vi "FOCUS_V42_H37.vi"(9 "X-pixels":sgl=256.0, 11 "Run":bool) -> (0 "Retrace pixels":sgl, 10 "Pixel Clock (Hz)":sgl)   [LabVIEW 2010] (continued)
                      tunnel: w5384 -> [w5402 w5420]
                      tunnel: w5353 -> [w5401 w5419]
                      tunnel: [w5400 w5418] -> w5383
                      tunnel: [w5399 w5417] -> w5382
                      tunnel: [w5399 w5417] -> w5369
                      tunnel: w5368 -> [_ _]
                      tunnel: w5361 -> [w5398 _]
                      tunnel: w5360 -> [w5394 w5415]
                      tunnel: [w5396 w5413] -> w5342
                      tunnel: w5341 -> [w5395 _]
                      frame False {
                        n2973 = case shown="True" w5395 {
                          tunnel: [w5403 w5404] -> w5396
                          tunnel: w5394 -> [w5403 _]
                          frame False {
                          }
                          frame True {
                            n2974 = local read "scattering length [µm]"() -> (w5412:sgl)
                            n2975 = local read "z-step (um)"() -> (w5408:sgl)
                            n2976 = Divide(x=w5408, y=w5412) -> (x/y=w5409:sgl)
                            n2977 = Exponential(1:w5409) -> (0:w5410:sgl)
                            n2978 = local read "Intensity"() -> (w5411:sgl)
                            n2979 = local read "IntensityScaleMax"() -> (w5405:sgl)
                            n2980 = Multiply(x=w5411, y=w5410) -> (x*y=w5406:sgl)
                            n2981 = In Range and Coerce(upper limit=sgl 0.0, x=w5406, lower limit=w5405) -> (coerced(x)=w5404:sgl)  [unwired: 1 out]
                            n2982 = local write "Intensity"(w5404) -> ()
                          }
                        }
                        n2983 = Build Array(w5398, w5396) -> (w5397:dbl[])
                        n2984 = call-poly <vilib>:"DAQmx Write (Analog 1D DBL NChan 1Samp).vi"("task/channels in"=w5402, "data"=w5397, "error in"=w5401) -> ("task out"=w5399:refnum<k21>, "error out"=w5400:errorcluster)  [unwired: 10 in, 1 out]
                      }
                      frame True {
                        n2985 = local read "IntensityScaleMax"() -> (w5414:sgl)
                        n2986 = In Range and Coerce(upper limit=sgl 0.0, x=w5415, lower limit=w5414) -> (coerced(x)=w5413:sgl)  [unwired: 1 out]
                        n2987 = local write "Intensity"(w5413) -> ()
                        n2988 = Build Array(0.0 ("data"), w5413) -> (w5422:dbl[])
                        n2989 = call-poly <vilib>:"DAQmx Write (Analog 1D DBL NChan 1Samp).vi"("task/channels in"=w5420, "data"=w5422, "error in"=w5419) -> ("task out"=w5417:refnum<k21>, "error out"=w5418:errorcluster)  [unwired: 10 in, 1 out]
                      }
                    }
                    n2990 = case shown="False" w5327 {
                      tunnel: [w5432 w5458] -> w5372
                      tunnel: [w5431 w5457] -> w5371
                      tunnel: [w5429 w5455] -> w5357
                      tunnel: w5370 -> [w5428 w5458]
                      tunnel: w5369 -> [w5427 _]
                      tunnel: w5368 -> [w5426 w5457]
                      tunnel: w5359 -> [w5425 w5456]
                      tunnel: [w5424 w5456] -> w5358
                      tunnel: w5363 -> [w5423 w5455]
                      frame False {
                        n2991 = flat-sequence {
                          tunnel: sgl 100.0 ("Time interval [s]") -> [w5444]
                          tunnel: [w5444] -> w5438
                          tunnel: [w5440] -> w5437
                          tunnel: [w5439] -> w5436
                          tunnel: w5428 -> [w5442]
                          tunnel: w5426 -> [w5441]
                          tunnel: [w5451] -> w5435
                          tunnel: [w5450] -> w5434
                          tunnel: [w5449] -> w5433
                          tunnel: w5438 -> [w5451]
                          tunnel: w5437 -> [w5450]
                          tunnel: w5436 -> [w5449]
                          tunnel: w5425 -> [w5448]
                          tunnel: w5423 -> [w5447]
                          tunnel: [w5446] -> w5429
                          tunnel: [w5445] -> w5424
                          tunnel: [w5454] -> w5432
                          tunnel: w5435 -> [w5453]
                          tunnel: w5434 -> [w5454]
                          tunnel: w5433 -> [w5452]
                          tunnel: [w5452] -> w5431
                          tunnel: w5427 -> [_]
                          frame #0 {
                            w5443 = FALSE ("data")
                            n2992 = local write "Shutter open"(w5443) -> ()
                            n2993 = call-poly <vilib>:"DAQmx Write (Digital Bool 1Line 1Point).vi"("task/channels in"=w5442, "data"=w5443, "error in"=w5441) -> ("task out"=w5440:refnum<k21>, "error out"=w5439:errorcluster)  [unwired: 10 in, 1 out]
                          }
                          frame #1 {
                            n2994 = call <vilib>:"DAQmx Stop Task.vi"("task/channels in"=w5448, "error in"=w5447) -> ("task out"=w5445:refnum<k21>, "error out"=w5446:errorcluster)  [unwired: 12 in]
                          }
                          frame #2 {
                            n2995 = Wait (ms)(milliseconds to wait=w5453) -> ()  [unwired: 1 out]
                          }
                        }
                      }
                      frame True {
                      }
                    }
                    n2996 = call "ConvertImagesDataFOCUS.vi"("Save mode"=w5321, "Image3"=w5325, "Image2"=w5334, "Image1"=w5335) -> ("Data"=w5333:u8[])
                    n2997 = Set File Position(refnum=w5339, from (0:start)=enum16{"start", "end", "current"}."current" ("pos mode (0:2)"), error in=w5338) -> (refnum out=w5320:refnum<file>, error out=w5319:errorcluster)  [unwired: 1 in]
                    n2998 = Write to Binary File(file (use dialog)=w5320, data=w5333, error in=w5319, 5:FALSE ("prepend array or string size? (T)")) -> (refnum out=w5337:refnum<file>, error out=w5336:errorcluster)  [unwired: 2 in, 1 out]
                    n2999 = local read "Y-lines"() -> (w5381:sgl)
                    n3000 = Multiply(x=w5354, y=w5381) -> (x*y=w5379:sgl)
                    n3001 = Replace Array Subset(array=w5386, new element=w5335, index (row)=0 ("disabled index (row)"), index (col)=w5379) -> (w5385:u8[][])
                    n3002 = Replace Array Subset(array=w5388, new element=w5334, index (row)=0 ("disabled index (row)"), index (col)=w5379) -> (w5387:u8[][])
                  }
                  n3003 = Not Equal?(x=w5254, y=w5255) -> (x != y?=w5256:bool)
                  n3004 = local write "IntDevUsed"(w5256) -> ()
                  n3005 = Close File(refnum=w5241, error in=w5240) -> ()  [unwired: 2 out]
                  n3006 = flat-sequence {
                    tunnel: [w5303] -> w5265
                    tunnel: w5267 -> [w5303]
                    tunnel: w5266 -> [w5302]
                    tunnel: [w5302] -> w5264
                    frame #0 {
                      n3007 = Tick Count (ms)() -> (millisecond timer value=w5304:u32)
                      n3008 = local write "stop"(w5304) -> ()
                    }
                  }
                }
                frame 5 {
                  w5745 = sgl 1000000.0 ("y")
                  w5777 = 0.0 ("X Scale.Range:Minimum")
                  w5784 = TRUE ("Visible")
                  # "User-defined line 3D"
                  n3009 = Greater Or Equal?(x=w5711, y=u16 3) -> (x >= y?=w5709:bool)
                  n3010 = property on="Property Node" class="VI"() -> ("VI Path"=w5739:path)  [unwired: 2 in, 2 out]
                  n3011 = property on="Property Node" class="VI"() -> ("VI Path"=w5720:path)  [unwired: 2 in, 2 out]
                  n3012 = flat-sequence {
                    tunnel: w5786 -> [w5801]
                    tunnel: [w5801] -> w5785
                    frame #0 {
                      n3013 = Tick Count (ms)() -> (millisecond timer value=w5802:u32)
                      n3014 = local write "start"(w5802) -> ()
                    }
                  }
                  n3015 = Unbundle By Name(w5724) -> ("status"=w5758:bool)
                  n3016 = Increment(x=w5735) -> (x+1=w5734:sgl)
                  n3017 = Tick Count (ms)() -> (millisecond timer value=w5790:u32)
                  n3018 = Strip Path(path=w5739) -> (stripped path=w5738:path)  [unwired: 1 out]
                  n3019 = Strip Path(path=w5720) -> (stripped path=w5719:path)  [unwired: 1 out]
                  n3020 = local read "X-pixels FreeLine"() -> (w5744:sgl)
                  n3021 = local read "Y-lines FreeLine"() -> (w5746:sgl)
                  n3022 = Build Path(base path=w5738, name or relative path="FreeLine.tmp") -> (appended path=w5737:path)
                  n3023 = Build Path(base path=w5719, name or relative path="EEG.tmp") -> (appended path=w5718:path)
                  n3024 = call <vilib>:"Open_Create_Replace File.vi"("advisory dialog? (display:T)"=FALSE, "function (open:0)"=T8."create or replace", "file path"=w5737) -> ("error out"=w5728:errorcluster, "refnum"=w5730:refnum<file>)  [unwired: 5 in, 2 out]
                  n3025 = Unbundle By Name(w5760) -> ("status"=w5759:bool)
                  n3026 = call <vilib>:"Open_Create_Replace File.vi"("advisory dialog? (display:T)"=FALSE, "function (open:0)"=T8."create or replace", "file path"=w5718) -> ("error out"=w5716:errorcluster, "refnum"=w5715:refnum<file>)  [unwired: 5 in, 2 out]
                  n3027 = Divide(x=w5745, y=w5744) -> (x/y=w5743:sgl)
                  n3028 = Multiply(x=w5746, y=w5744) -> (x*y=w5747:sgl)
                  n3029 = local read "XScale"() -> (w5778:bool)
                  n3030 = Greater?(x=w5747, y=w5745) -> (0:w5748:bool)
                  n3031 = Select(t=w5743, s=w5748, f=w5746) -> (s? t:f=w5742:sgl)
                  n3032 = case shown="True" w5778 {
                    tunnel: [w5797 w5798] -> w5776
                    tunnel: w5742 -> [w5797 _]
                    tunnel: w5744 -> [_ w5798]
                    frame False {
                    }
                    frame True {
                    }
                  }
                  n3033 = Set File Position(refnum=w5730, from (0:start)=enum16{"start", "end", "current"}."start" ("pos mode (rel. to end:1)"), error in=w5728) -> (refnum out=w5708:refnum<file>, error out=w5707:errorcluster)  [unwired: 1 in]
                  n3034 = Write to Binary File(file (use dialog)=w5708, data=w5731, error in=w5707, 5:FALSE ("prepend array or string size? (T)")) -> (refnum out=w5729:refnum<file>, error out=w5727:errorcluster)  [unwired: 2 in, 1 out]
                  n3035 = while {
                    tunnel: [w5842] -> w5791
                    tunnel: [w5840] -> w5788
                    tunnel: w5792 -> [w5871]
                    tunnel: w5785 -> [w5864]
                    shift-right: [w5847] -> w5752
                    shift-left: w5793 -> [w5903]
                    tunnel: w5749 -> [w5818]
                    shift-right: [w5849] -> w5753
                    shift-left: w5793 -> [w5902]
                    shift-right: [w5897] -> _
                    shift-left: w5790 -> [w5898]
                    tunnel: w5782 -> [w5874]
                    tunnel: w5781 -> [w5865]
                    tunnel: [w5873] -> w5779
                    tunnel: [w5872] -> w5780
                    shift-right: [w5877] -> w5733
                    shift-left: w5775 -> [w5879]
                    tunnel: w5765 -> [w5875]
                    tunnel: w5764 -> [w5863]
                    tunnel: [w5875] -> w5762
                    tunnel: [w5863] -> w5763
                    tunnel: [w5867] -> w5761
                    tunnel: w5759 -> [w5862]
                    tunnel: w5758 -> [w5858]
                    shift-right: [w5851] -> w5750
                    shift-left: w5729 -> [w5853]
                    shift-right: [w5850] -> w5751
                    shift-left: w5727 -> [w5852]
                    tunnel: w5734 -> [w5844]
                    tunnel: w5726 -> [w5838]
                    tunnel: w5724 -> [w5837]
                    tunnel: [w5836] -> w5725
                    tunnel: [w5835] -> w5723
                    shift-right: [w5827] -> w5714
                    shift-left: w5715 -> [w5829]
                    shift-right: [w5826] -> w5713
                    shift-left: w5716 -> [w5828]
                    tunnel: w5712 -> [w5824]
                    tunnel: w5711 -> [w5814]
                    tunnel: w5709 -> [w5809]
                    i -> [w5845]
                    stop <- w5854 stop-if-true
                    # "DIO Read reads one\nline of data at a time"
                    n3036 = Unbundle By Name(w5863) -> ("status"=w5861:bool)
                    n3037 = Unbundle By Name(w5865) -> ("status"=w5860:bool)
                    n3038 = Equal To 0?(x=w5845) -> (x = 0?=w5884:bool)
                    n3039 = Unbundle By Name(w5864) -> ("status"=w5859:bool)
                    n3040 = local read "End experiment"() -> (w5856:bool)
                    n3041 = local read "Y-lines FreeLine"() -> (w5866:sgl)
                    n3042 = case shown="False" w5884 {
                      tunnel: w5818 -> [w5963 w5966]
                      tunnel: [w5963 w5965] -> w5817
                      tunnel: w5824 -> [_ w5964]
                      tunnel: [sgl 0.0 w5964] -> w5819
                      frame False {
                      }
                      frame True {
                        n3043 = Add(x=w5966, y=w5964) -> (x+y=w5965:sgl)
                      }
                    }
                    n3044 = call-poly <vilib>:"DAQmx Read (Analog 2D DBL NChan NSamp).vi"("task/channels in"=w5874, "number of samples per channel"=w5817, "error in"=w5865) -> ("task out"=w5873:refnum<k21>, "data"=w5821:dbl[][], "error out"=w5872:errorcluster)  [unwired: 10 in]
                    n3045 = Array Subset(array=w5821, index (col)=w5819) -> (w5820:dbl[][])  [unwired: 3 in]
                    n3046 = local read "stop 2"() -> (w5857:bool)
                    n3047 = Transpose 2D Array(2D array=w5820) -> (transposed array=w5831:dbl[][])
                    n3048 = Increment(x=w5845) -> (x+1=w5876:i32)
                    n3049 = call-poly <vilib>:"DAQmx Read (Digital 1D U32 1Chan NSamp).vi"("task/channels in"=w5871, "number of samples per channel"=w5817, "error in"=w5864) -> ("task out"=w5843:refnum<k21>, "data"=w5823:u32[], "error out"=w5841:errorcluster)  [unwired: 10 in]
                    n3050 = Build Array (concatenate)(w5879, w5831) -> (w5878:dbl[][])
                    n3051 = Multiply(x="z frequency", y=w5818) -> (x*y=w5834:dbl)
                    n3052 = Index Array(array=w5831, index (col)=0 ("disabled index (col)")) -> (element=w5881:dbl[])  [unwired: 1 in]
                    n3053 = Equal?(x=w5876, y=w5866) -> (x = y?=w5855:bool)
                    n3054 = local write "#"(w5876) -> ()
                    n3055 = Index Array(array=w5831, index (col)=1 ("disabled index (col)")) -> (element=w5880:dbl[])  [unwired: 1 in]
                    n3056 = Array Subset "Extract DI0"(array=w5823, index=w5819) -> (w5822:u32[])  [unwired: 1 in]
                    n3057 = Index Array(array=w5831, index (col)=3 ("disabled index (col)")) -> (element=w5825:dbl[])  [unwired: 1 in]
                    n3058 = local read "Overlay Images"() -> (w5885:bool)
                    n3059 = property class="DAQmx Timing"(reference=w5838, error in=w5837, "Sample Clock:Rate"=w5834) -> (reference out=w5836:refnum<k21>, error out=w5835:errorcluster)
                    n3060 = Compound Arithmetic op=OR(w5855, w5856, w5857, w5858, w5859, w5860, w5861, w5862) -> (w5854:bool)
                    n3061 = Array Subset(array=w5878, index (row)=w5818) -> (w5877:dbl[][])  [unwired: 3 in]
                    n3062 = local read "x scale"() -> (w5891:dbl)
                    n3063 = local read "y scale"() -> (w5889:dbl)
                    n3064 = Split Number(x=w5822) -> (hi(x)=w5816:u16[], lo(x)=w5815:u16[])
                    n3065 = property class="DAQmx Read"(reference=w5843, error in=w5841) -> (reference out=w5842:refnum<k21>, error out=w5840:errorcluster, "Status:Available Samples Per Channel"=→"Scan Backlock":u32)
                    n3066 = case shown="0, Default" w5814 {
                      tunnel: w5816 -> [w5915 w5920 w5925 w5930 w5935 w5940]
                      tunnel: [w5914 w5919 w5922 w5929 w5934 w5937] -> w5813
                      tunnel: [w5912 w5917 w5924 w5927 w5932 w5939] -> w5812
                      tunnel: w5815 -> [w5913 w5918 w5923 w5928 w5933 w5938]
                      tunnel: [w5911 w5916 w5921 w5926 w5931 w5936] -> w5811
                      frame 0, Default {
                        n3067 = Split Number(x=w5915) -> (hi(x)=w5914:u8[], lo(x)=w5912:u8[])
                        n3068 = Split Number(x=w5913) -> (lo(x)=w5911:u8[])  [unwired: 1 out]
                      }
                      frame 1 {
                        n3069 = Split Number(x=w5920) -> (hi(x)=w5919:u8[], lo(x)=w5916:u8[])
                        n3070 = Split Number(x=w5918) -> (lo(x)=w5917:u8[])  [unwired: 1 out]
                      }
                      frame 2 {
                        n3071 = Split Number(x=w5925) -> (hi(x)=w5921:u8[], lo(x)=w5924:u8[])
                        n3072 = Split Number(x=w5923) -> (lo(x)=w5922:u8[])  [unwired: 1 out]
                      }
                      frame 3 {
                        n3073 = Split Number(x=w5930) -> (hi(x)=w5929:u8[], lo(x)=w5927:u8[])
                        n3074 = Split Number(x=w5928) -> (lo(x)=w5926:u8[])  [unwired: 1 out]
                      }
                      frame 4 {
                        n3075 = Split Number(x=w5935) -> (hi(x)=w5934:u8[], lo(x)=w5931:u8[])
                        n3076 = Split Number(x=w5933) -> (lo(x)=w5932:u8[])  [unwired: 1 out]
                      }
                      frame 5 {
                        n3077 = Split Number(x=w5940) -> (hi(x)=w5936:u8[], lo(x)=w5939:u8[])
                        n3078 = Split Number(x=w5938) -> (lo(x)=w5937:u8[])  [unwired: 1 out]
                      }
                    }
                    n3079 = Tick Count (ms)() -> (millisecond timer value=w5899:u32)
                    n3080 = Multiply(x=w5880, y=w5889) -> (x*y=w5893:dbl[])
                    n3081 = Multiply(x=w5891, y=w5881) -> (x*y=w5895:dbl[])
                    n3082 = local read "x offset"() -> (w5890:dbl)
                    n3083 = case shown="True" w5885 {
                      tunnel: w5813 -> [w5968 w5971]
                      tunnel: [w5968 w5969] -> w5887
                      tunnel: w5812 -> [w5967 w5970]
                      tunnel: [w5967 _] -> w5886
                      frame False {
                      }
                      frame True {
                        n3084 = To Word Integer(number=w5971) -> (16bit integer=w5976:i16[])
                        n3085 = Subtract(x=w5976, y=w5970) -> (x-y=w5977:i16[])
                        n3086 = Add(x=w5976, y=w5970) -> (x+y=w5981:i16[])
                        n3087 = Increment(x=w5981) -> (x+1=w5972:i16[])
                        n3088 = Divide(x=w5977, y=w5972) -> (x/y=w5973:dbl[])
                        n3089 = Absolute Value(x=w5977) -> (abs(x)=w5979:i16[])
                        n3090 = Multiply(x=w5973, y=u8 2) -> (x*y=w5975:dbl[])
                        n3091 = Round To Nearest(number=w5975) -> (nearest integer value=w5988:dbl[])
                        n3092 = Divide(x=w5979, y=2.0) -> (x/y=w5982:dbl[])
                        n3093 = Divide(x=w5981, y=2.0) -> (x/y=w5983:dbl[])
                        n3094 = Add(x=w5982, y=w5983) -> (x+y=w5985:dbl[])
                        n3095 = Divide(x=w5985, y=5.0) -> (x/y=w5986:dbl[])
                        n3096 = Round To Nearest(number=w5986) -> (nearest integer value=w5987:dbl[])
                        n3097 = Multiply(x=5.0 ("y"), y=w5987) -> (x*y=w5989:dbl[])
                        n3098 = Add(x=w5988, y=w5989) -> (x+y=w5990:dbl[])
                        n3099 = Subtract(x=w5990, y=2.0) -> (x-y=w5993:dbl[])
                        n3100 = To Unsigned Byte Integer(number=w5993) -> (unsigned 8bit integer=w5969:u8[])
                      }
                    }
                    n3101 = Subtract(x=w5899, y=w5898) -> (x-y=w5900:u32)
                    n3102 = local read "y offset"() -> (w5888:dbl)
                    n3103 = local read "Image Update [ms]"() -> (w5870:u32)
                    n3104 = Add(x=w5893, y=w5888) -> (x+y=w5892:dbl[])
                    n3105 = Add(x=w5890, y=w5895) -> (x+y=w5894:dbl[])
                    n3106 = Subtract(x=w5845, y=w5818) -> (x-y=w5867:sgl)
                    n3107 = case shown="True" w5809 {
                      tunnel: w5813 -> [w5907 w5910]
                      tunnel: w5812 -> [w5904 w5909]
                      tunnel: w5811 -> [w5906 _]
                      tunnel: [w5905 w5908] -> w5810
                      frame True {
                        n3108 = Interleave 1D Arrays(w5904, w5907, w5906) -> (w5905:u8[])
                      }
                      frame False {
                        n3109 = Interleave 1D Arrays(w5910, w5909) -> (w5908:u8[])
                      }
                    }
                    n3110 = Multiply(x=w5870, y=u32 20) -> (x*y=w5868:u32)
                    n3111 = Greater Or Equal?(x=w5900, y=w5868) -> (x >= y?=w5901:bool)
                    n3112 = Greater Or Equal?(x=w5845, y=w5844) -> (x >= y?=w5846:bool)
                    n3113 = case shown="True" w5846 {
                      tunnel: w5903 -> [w5947 w5960]
                      tunnel: w5902 -> [w5946 w5954]
                      tunnel: w5887 -> [w5945 w5958]
                      tunnel: w5886 -> [w5944 w5951]
                      tunnel: [w5943 w5948] -> w5849
                      tunnel: [w5942 w5961] -> w5847
                      tunnel: w5845 -> [w5941 _]
                      frame False {
                        n3114 = Replace Array Subset(array=w5947, new element=w5945, index (col)=w5941) -> (w5942:u8[][])  [unwired: 1 in]
                        n3115 = Replace Array Subset(array=w5946, new element=w5944, index (col)=w5941) -> (w5943:u8[][])  [unwired: 1 in]
                      }
                      frame True {
                        n3116 = Transpose 2D Array(2D array=w5954) -> (transposed array=w5952:u8[][])
                        n3117 = Transpose 2D Array(2D array=w5960) -> (transposed array=w5959:u8[][])
                        n3118 = Build Array (concatenate)(w5952, w5951) -> (w5953:u8[][])
                        n3119 = Build Array (concatenate)(w5959, w5958) -> (w5957:u8[][])
                        n3120 = Transpose 2D Array(2D array=w5953) -> (transposed array=w5949:u8[][])
                        n3121 = Transpose 2D Array(2D array=w5957) -> (transposed array=w5956:u8[][])
                        n3122 = Array Subset(array=w5956, index (col)=1 ("index")) -> (w5961:u8[][])  [unwired: 3 in]
                        n3123 = Array Subset(array=w5949, index (col)=1 ("index")) -> (w5948:u8[][])  [unwired: 3 in]
                      }
                    }
                    n3124 = Set File Position(refnum=w5829, from (0:start)=enum16{"start", "end", "current"}."current" ("pos mode (0:2)"), error in=w5828) -> (refnum out=w5808:refnum<file>, error out=w5807:errorcluster)  [unwired: 1 in]
                    n3125 = Write to Binary File(file (use dialog)=w5808, data=w5825, error in=w5807, 5:FALSE ("prepend array or string size? (T)")) -> (refnum out=w5827:refnum<file>, error out=w5826:errorcluster)  [unwired: 2 in, 1 out]
                    n3126 = Set File Position(refnum=w5853, from (0:start)=enum16{"start", "end", "current"}."current" ("pos mode (0:2)"), error in=w5852) -> (refnum out=w5805:refnum<file>, error out=w5804:errorcluster)  [unwired: 1 in]
                    n3127 = Write to Binary File(file (use dialog)=w5805, data=w5810, error in=w5804, 5:FALSE ("prepend array or string size? (T)")) -> (refnum out=w5851:refnum<file>, error out=w5850:errorcluster)  [unwired: 2 in, 1 out]
                    n3128 = Bundle(w5894, w5892) -> (w5896:cluster{dbl[], dbl[]})  [unwired: 1 in]
                    n3129 = case shown="True" w5901 {
                      tunnel: [w5994 w5998] -> w5897
                      tunnel: w5898 -> [w5994 _]
                      tunnel: w5896 -> [_ w5997]
                      tunnel: w5847 -> [_ w5996]
                      tunnel: w5849 -> [_ w5995]
                      frame False {
                      }
                      frame True {
                        n3130 = local write "XY Graph 3"(w5997) -> ()
                        n3131 = local write "XY Graph 4"(w5997) -> ()
                        n3132 = local write "Image 4"(w5995) -> ()
                        n3133 = local write "Image 3"(w5996) -> ()
                        n3134 = Tick Count (ms)() -> (millisecond timer value=w5998:u32)
                      }
                    }
                  }
                  n3135 = property on="Image 2" class="IntGraph (strict)"() -> ("Color Table"=w5783:u32[])  [unwired: 2 in, 2 out]
                  n3136 = property on="Image 3" class="IntGraph (strict)"("X Scale.Range:Minimum"=w5777, "X Scale.Range:Maximum"=w5776, "Y Scale.Range:Minimum"=w5777, "Y Scale.Range:Maximum"=w5742, "Visible"=w5784, "Color Table"=w5783) -> ()  [unwired: 2 in, 2 out]
                  n3137 = property on="Image 4" class="IntGraph (strict)"("X Scale.Range:Minimum"=w5777, "X Scale.Range:Maximum"=w5776, "Y Scale.Range:Minimum"=w5777, "Y Scale.Range:Maximum"=w5742, "Visible"=w5784, "Color Table"=w5783) -> ()  [unwired: 2 in, 2 out]
                  n3138 = property on="Histogram1" class="XYGraph (strict)"("X Scale.Range:Minimum"=w5777, "X Scale.Range:Maximum"=w5776) -> ()  [unwired: 2 in, 2 out]
                  n3139 = property on="Histogram2" class="XYGraph (strict)"("X Scale.Range:Minimum"=w5777, "X Scale.Range:Maximum"=w5776) -> ()  [unwired: 2 in, 2 out]
                  n3140 = Close File(refnum=w5750, error in=w5751) -> ()  [unwired: 2 out]
                  n3141 = Close File(refnum=w5714, error in=w5713) -> ()  [unwired: 2 out]
                  n3142 = Array Subset(array=w5733, index (col)=0 ("index"), length (col)=3 ("length")) -> (w5766:dbl[][])  [unwired: 2 in]
                  n3143 = Index Array(array=w5766, index (col)=0 ("disabled index (col)")) -> (element=w5773:dbl[])  [unwired: 1 in]
                  n3144 = flat-sequence {
                    tunnel: w5788 -> [w5799]
                    tunnel: [w5799] -> w5787
                    frame #0 {
                      n3145 = Tick Count (ms)() -> (millisecond timer value=w5800:u32)
                      n3146 = local write "stop"(w5800) -> ()
                    }
                  }
                  n3147 = Array Size(array=w5773) -> (size(s)=w5772:i32)
                  n3148 = Multiply(x=w5772, y=3) -> (x*y=w5770:i32)
                  n3149 = Reshape Array(w5766, w5770) -> (w5769:dbl[])
                  n3150 = local write "Positions"(w5769) -> ()
                }
              }
            }
            frame True {
              n3151 = local read "scans to read"() -> (w6008:sgl)
              n3152 = local read "Number of Frames"() -> (w6005:sgl)
              n3153 = Multiply(x=w6008, y=w6007) -> (x*y=w6004:sgl)
              n3154 = Multiply(x=w6006, y=w6005) -> (x*y=w6011:sgl)
              n3155 = Reciprocal(x=w6004) -> (1/x=w6003:sgl)
              n3156 = local write "Frame rate [Hz]"(w6003) -> ()
              n3157 = case shown="0, Default" w6051 {
                tunnel: w6050 -> [w6085 w6320 w6508]
                tunnel: w6049 -> [w6086 w6321 w6509]
                tunnel: w6048 -> [w6074 w6309 w6497]
                tunnel: w6047 -> [w6084 w6319 w6507]
                tunnel: w6046 -> [w6073 w6308 w6496]
                tunnel: w6045 -> [w6079 w6314 w6502]
                tunnel: w6044 -> [w6078 w6313 w6501]
                tunnel: w6043 -> [w6083 w6318 w6506]
                tunnel: w6042 -> [w6082 w6317 w6505]
                tunnel: w6041 -> [w6088 w6299 w6487]
                tunnel: w6040 -> [w6069 w6298 w6486]
                tunnel: w6039 -> [w6089 w6323 w6511]
                tunnel: w6038 -> [w6070 w6305 w6493]
                tunnel: w6037 -> [w6090 w6324 w6512]
                tunnel: [w6090 w6324 w6512] -> w6036
                tunnel: [w6070 w6305 w6493] -> w6034
                tunnel: [w6089 w6323 w6511] -> w6035
                tunnel: [w6069 w6296 w6484] -> w6032
                tunnel: [w6088 w6297 w6485] -> w6033
                tunnel: [768 ("DataOffset") 768 ("DataOffset") 768 ("DataOffset")] -> w6031
                tunnel: [0 ("DataOffset") 0 ("DataOffset") 0 ("DataOffset")] -> w6030
                tunnel: [0 ("DataOffset") 0 ("DataOffset") 0 ("DataOffset")] -> w6029
                tunnel: [w6080 w6315 w6503] -> w6028
                tunnel: [w6081 w6316 w6504] -> w6027
                tunnel: [w6076 w6311 w6499] -> w6026
                tunnel: [w6077 w6312 w6500] -> w6025
                tunnel: [w6074 w6309 w6497] -> w6024
                tunnel: [w6086 w6321 w6509] -> w6023
                tunnel: [w6085 w6320 w6508] -> w6022
                tunnel: [w6073 w6308 w6496] -> w6021
                tunnel: [w6084 w6319 w6507] -> w6020
                tunnel: w6019 -> [w6056 w6284 w6498]
                tunnel: w6018 -> [w6063 w6302 w6490]
                tunnel: w6008 -> [_ w6291 w6483]
                tunnel: w6017 -> [w6062 w6290 w6482]
                tunnel: w6016 -> [w6061 w6289 w6481]
                tunnel: w6015 -> [w6060 w6287 w6479]
                tunnel: w6014 -> [w6059 w6288 w6480]
                tunnel: [w6058 w6287 w6479] -> w6013
                tunnel: [w6057 w6288 w6480] -> w6012
                tunnel: w6011 -> [_ w6286 _]
                tunnel: w6010 -> [_ w6285 _]
                tunnel: [_ w6282 w6474] -> w6009
                tunnel: w6007 -> [w6054 _ _]
                tunnel: [w6053 w6280 w6473] -> w6002
                tunnel: [w6052 w6279 w6472] -> w6001
                frame 0, Default {
                  # "Focus mode FScope"
                  n3158 = To Unsigned Long Integer(number=w6056) -> (unsigned 32bit integer=w6055:u32[][])
                  n3159 = Tick Count (ms)() -> (millisecond timer value=w6075:u32)
                  n3160 = Unbundle By Name(w6074) -> ("status"=w6072:bool)
                  n3161 = Unbundle By Name(w6073) -> ("status"=w6071:bool)
                  n3162 = Unbundle By Name(w6069) -> ("status"=w6068:bool)
                  n3163 = Unbundle By Name(w6070) -> ("status"=w6067:bool)
                  n3164 = while {
                    tunnel: w6083 -> [w6168]
                    tunnel: w6082 -> [w6167]
                    tunnel: [w6166] -> w6081
                    tunnel: [w6155] -> w6080
                    shift-right: [w6145] -> w6053
                    shift-left: w6056 -> [w6135]
                    shift-right: [w6116] -> w6052
                    shift-left: w6056 -> [w6132]
                    tunnel: [w6160] -> w6077
                    tunnel: w6079 -> [w6160]
                    tunnel: [w6156] -> w6076
                    tunnel: w6078 -> [w6156]
                    shift-right: [w6143] -> _
                    shift-left: w6075 -> [w6144]
                    shift-right: [w6098] -> _
                    shift-left: w6055 -> [w6138]
                    tunnel: w6072 -> [w6152]
                    tunnel: w6071 -> [w6157]
                    tunnel: w6068 -> [w6151]
                    tunnel: w6067 -> [w6150]
                    shift-right: [w6141] -> _
                    shift-left: 0.0 ("millisecond timer value") -> [w6120]
                    tunnel: w6063 -> [w6140]
                    shift-right: [w6123] -> _
                    shift-left: w6061 -> [w6125]
                    shift-right: [w6122] -> _
                    shift-left: w6062 -> [w6124]
                    tunnel: w6060 -> [w6104]
                    tunnel: w6059 -> [w6103]
                    tunnel: [w6102] -> w6058
                    tunnel: [w6101] -> w6057
                    tunnel: w6054 -> [w6094]
                    stop <- w6149 stop-if-true
                    n3165 = Multiply(x="scans to read", y=w6094) -> (x*y=w6092:sgl)
                    n3166 = Bundle("ScaleCluster"="ScaleCluster", "scans to read"="scans to read") -> (w6123:T20)  [unwired: 1 in]
                    n3167 = Reciprocal(x=w6092) -> (1/x=→"Frame rate [Hz]":sgl)
                    n3168 = call-poly <vilib>:"DAQmx Read (Digital 1D U32 1Chan NSamp).vi"("task/channels in"=w6168, "number of samples per channel"="scans to read", "error in"=w6167) -> ("task out"=w6166:refnum<k21>, "data"=w6096:u32[], "error out"=w6155:errorcluster)  [unwired: 10 in]
                    n3169 = local read "Overlay Images"() -> (w6163:bool)
                    n3170 = Not Equal?(x=w6123, y=w6125) -> (x != y?=w6126:bool)
                    n3171 = Multiply(x=u32 0 ("millisecond timer value"), y=w6138) -> (x*y=w6137:u32[][])
                    n3172 = case shown="True" w6126 {
                      tunnel: w6140 -> [_ w6247]
                      tunnel: w6123 -> [_ w6246]
                      tunnel: [w6244 w6245] -> w6122
                      tunnel: w6124 -> [w6244 _]
                      frame False {
                      }
                      frame True {
                        n3173 = call "ScaleScanlineFScope.vi"("Parameters"=w6247, "ScaleCluster"=w6246) -> ("ScanlineScaled"=w6245:dbl[][])
                      }
                    }
                    n3174 = Split Number(x=w6096) -> (hi(x)=w6165:u16[])  [unwired: 1 out]
                    n3175 = Multiply(x=u8 0 ("millisecond timer value"), y=w6135) -> (x*y=w6134:u8[][])
                    n3176 = Split Number(x=w6165) -> (hi(x)=w6111:u8[], lo(x)=w6164:u8[])
                    n3177 = call-poly <vilib>:"Ramp Pattern.vi"("start"=0.0, "end"=6.283185307179586, "samples"="scans to read") -> ("Ramp Pattern"=w6115:dbl[])  [unwired: 7 in, 1 out]
                    n3178 = case shown="True" w6163 {
                      tunnel: w6111 -> [w6253 w6272]
                      tunnel: [w6253 w6255] -> w6147
                      tunnel: w6164 -> [w6252 w6274]
                      tunnel: [w6252 _] -> w6146
                      frame False {
                      }
                      frame True {
                        n3179 = To Word Integer(number=w6272) -> (16bit integer=w6273:i16[])
                        n3180 = Subtract(x=w6273, y=w6274) -> (x-y=w6254:i16[])
                        n3181 = Add(x=w6273, y=w6274) -> (x+y=w6268:i16[])
                        n3182 = Increment(x=w6268) -> (x+1=w6278:i16[])
                        n3183 = Divide(x=w6254, y=w6278) -> (x/y=w6277:dbl[])
                        n3184 = Absolute Value(x=w6254) -> (abs(x)=w6270:i16[])
                        n3185 = Multiply(x=w6277, y=u8 2) -> (x*y=w6275:dbl[])
                        n3186 = Round To Nearest(number=w6275) -> (nearest integer value=w6261:dbl[])
                        n3187 = Divide(x=w6270, y=2.0) -> (x/y=w6267:dbl[])
                        n3188 = Divide(x=w6268, y=2.0) -> (x/y=w6266:dbl[])
                        n3189 = Add(x=w6267, y=w6266) -> (x+y=w6264:dbl[])
                        n3190 = Divide(x=w6264, y=5.0) -> (x/y=w6263:dbl[])
                        n3191 = Round To Nearest(number=w6263) -> (nearest integer value=w6262:dbl[])
                        n3192 = Multiply(x=5.0 ("y"), y=w6262) -> (x*y=w6260:dbl[])
                        n3193 = Add(x=w6261, y=w6260) -> (x+y=w6259:dbl[])
                        n3194 = Subtract(x=w6259, y=2.0) -> (x-y=w6256:dbl[])
                        n3195 = To Unsigned Byte Integer(number=w6256) -> (unsigned 8bit integer=w6255:u8[])
                      }
                    }
                    n3196 = Multiply(x=u8 0 ("millisecond timer value"), y=w6132) -> (x*y=w6131:u8[][])
                    n3197 = Sine(x=w6115) -> (sin(x)=w6113:dbl[])
                    n3198 = Array Subset(array=w6122, index (col)=w6120, length (col)="scans to read") -> (w6127:dbl[][])  [unwired: 2 in]
                    n3199 = Add(x=w6113, y=sgl 2.0 ("millisecond timer value")) -> (x+y=w6107:dbl[])
                    n3200 = Index Array(array=w6122, index (row)=0) -> (element=w6129:dbl[])  [unwired: 1 in]
                    n3201 = Divide(x=u32 4294967295 ("millisecond timer value"), y=sgl 3.0) -> (x/y=w6108:sgl)
                    n3202 = Array Size(array=w6129) -> (size(s)=w6118:i32)
                    n3203 = Multiply(x=w6108, y=w6107) -> (x*y=w6106:dbl[])
                    n3204 = Add(x=w6120, y="scans to read") -> (x+y=w6128:dbl)
                    n3205 = Divide(x=w6118, y=2) -> (x/y=w6117:dbl)
                    n3206 = To Unsigned Long Integer(number=w6106) -> ()  [unwired: 1 out]
                    n3207 = Greater Or Equal?(x=w6128, y=w6117) -> (x >= y?=w6142:bool)
                    n3208 = case shown="True" w6142 {
                      tunnel: w6128 -> [w6248 w6251]
                      tunnel: [w6248 w6249] -> w6141
                      tunnel: w6117 -> [_ w6250]
                      frame False {
                      }
                      frame True {
                        n3209 = Subtract(x=w6251, y=w6250) -> (x-y=w6249:dbl)
                      }
                    }
                    n3210 = Tick Count (ms)() -> (millisecond timer value=w6162:u32)
                    n3211 = local read "Image Update [ms]"() -> (w6159:u32)
                    n3212 = call "AverageImageFScope.vi"("HitsArray"=w6137, "ScanLineFScope"=w6127, "Image1Array"=w6134, "Image2Array"=w6131, "DataImage2"=w6146, "DataImage1"=w6147) -> ("HitsArraynew"=w6098:u32[][], "Image1Arraynew"=w6145:u8[][], "Image2Arraynew"=w6116:u8[][])
                    n3213 = Subtract(x=w6162, y=w6144) -> (x-y=w6161:u32)
                    n3214 = Greater Or Equal?(x=w6161, y=w6159) -> ()  [unwired: 1 out]
                    n3215 = local write "Image 1"(w6145) -> ()
                    n3216 = local write "Image 2"(w6116) -> ()
                    n3217 = local write "Hit Graph"(w6098) -> ()
                    n3218 = Unbundle By Name(w6156) -> ("status"=w6154:bool)
                    n3219 = Unbundle By Name(w6155) -> ("status"=w6153:bool)
                    n3220 = event shown="[1] \"Up 100\": Mouse Down" {
                      selector: _ -> [_ _ _ _ _ _ _]
                      dyn-events: _ -> [_ _ _ _ _ _ _]
                      timeout: 0 -> [_ _ _ _ _ _ _]
                      tunnel: w6104 -> [w6170 w6183 w6195 w6207 w6219 w6231 w6243]
                      tunnel: w6103 -> [w6169 w6182 w6194 w6206 w6218 w6230 w6242]
                      tunnel: [w6170 w6178 w6190 w6202 w6214 w6226 w6238] -> w6102
                      tunnel: [w6169 w6177 w6189 w6201 w6213 w6225 w6237] -> w6101
                      tunnel: [w6171 w6172 w6184 w6196 w6210 w6222 w6234] -> w6099
                      event Timeout {
                        n3221 = event-data() -> ()  [unwired: 1 in, 2 out]
                        n3222 = global read "GlobelFSCOPE.vi" "Focus"() -> (w6171:dbl)
                      }
                      event "Up 100": Mouse Down {
                        n3223 = event-data() -> ()  [unwired: 1 in, 1 out]
                        n3224 = Multiply(x=100.0 ("y"), y=0.3763) -> (x*y=w6174:dbl)
                        n3225 = call "MotorDriveFOCUS.vi"("task in"=w6183, "interdelay (ms)"=i16 3, "Iterations"=100, "error in"=w6182, "Up / Down"=TRUE) -> ("task out"=w6178:refnum<k21>, "error out"=w6177:errorcluster)
                        n3226 = global read "GlobelFSCOPE.vi" "Focus"() -> (w6173:dbl)
                        n3227 = Add(x=w6174, y=w6173) -> (x+y=w6172:dbl)
                        n3228 = global write "GlobelFSCOPE.vi" "Focus"(w6172) -> ()
                      }
                      event "Up 10": Mouse Down {
                        n3229 = event-data() -> ()  [unwired: 1 in, 1 out]
                        n3230 = Multiply(x=10.0 ("y"), y=0.3763) -> (x*y=w6187:dbl)
                        n3231 = call "MotorDriveFOCUS.vi"("task in"=w6195, "interdelay (ms)"=i16 3, "Iterations"=10, "error in"=w6194, "Up / Down"=TRUE) -> ("task out"=w6190:refnum<k21>, "error out"=w6189:errorcluster)
                        n3232 = global read "GlobelFSCOPE.vi" "Focus"() -> (w6186:dbl)
                        n3233 = Add(x=w6187, y=w6186) -> (x+y=w6184:dbl)
                        n3234 = global write "GlobelFSCOPE.vi" "Focus"(w6184) -> ()
                      }
                      event "Up 1": Mouse Down {
                        n3235 = event-data() -> ()  [unwired: 1 in, 1 out]
                        n3236 = Multiply(x=1.0 ("y"), y=0.3763) -> (x*y=w6199:dbl)
                        n3237 = call "MotorDriveFOCUS.vi"("task in"=w6207, "interdelay (ms)"=i16 3, "Iterations"=1, "error in"=w6206, "Up / Down"=TRUE) -> ("task out"=w6202:refnum<k21>, "error out"=w6201:errorcluster)
                        n3238 = global read "GlobelFSCOPE.vi" "Focus"() -> (w6200:dbl)
                        n3239 = Add(x=w6199, y=w6200) -> (x+y=w6196:dbl)
                        n3240 = global write "GlobelFSCOPE.vi" "Focus"(w6196) -> ()
                      }
                      event "Down 100": Mouse Down {
                        n3241 = event-data() -> ()  [unwired: 1 in, 1 out]
                        n3242 = Multiply(x=100.0 ("y"), y=0.3763) -> (x*y=w6208:dbl)
                        n3243 = call "MotorDriveFOCUS.vi"("task in"=w6219, "interdelay (ms)"=i16 3, "Iterations"=100, "error in"=w6218, "Up / Down"=FALSE) -> ("task out"=w6214:refnum<k21>, "error out"=w6213:errorcluster)
                        n3244 = global read "GlobelFSCOPE.vi" "Focus"() -> (w6209:dbl)
                        n3245 = Subtract(x=w6209, y=w6208) -> (x-y=w6210:dbl)
                        n3246 = global write "GlobelFSCOPE.vi" "Focus"(w6210) -> ()
                      }
                      event "Down 10": Mouse Down {
                        n3247 = event-data() -> ()  [unwired: 1 in, 1 out]
                        n3248 = Multiply(x=10.0 ("y"), y=0.3763) -> (x*y=w6220:dbl)
                        n3249 = call "MotorDriveFOCUS.vi"("task in"=w6231, "interdelay (ms)"=i16 3, "Iterations"=10, "error in"=w6230, "Up / Down"=FALSE) -> ("task out"=w6226:refnum<k21>, "error out"=w6225:errorcluster)
                        n3250 = global read "GlobelFSCOPE.vi" "Focus"() -> (w6221:dbl)
                        n3251 = Subtract(x=w6221, y=w6220) -> (x-y=w6222:dbl)
                        n3252 = global write "GlobelFSCOPE.vi" "Focus"(w6222) -> ()
                      }
                      event "Down 1": Mouse Down {
                        n3253 = event-data() -> ()  [unwired: 1 in, 1 out]
                        n3254 = Multiply(x=1.0 ("y"), y=0.3763) -> (x*y=w6233:dbl)
                        n3255 = call "MotorDriveFOCUS.vi"("task in"=w6243, "interdelay (ms)"=i16 3, "Iterations"=1, "error in"=w6242, "Up / Down"=FALSE) -> ("task out"=w6238:refnum<k21>, "error out"=w6237:errorcluster)
                        n3256 = global read "GlobelFSCOPE.vi" "Focus"() -> (w6232:dbl)
                        n3257 = Subtract(x=w6232, y=w6233) -> (x-y=w6234:dbl)
                        n3258 = global write "GlobelFSCOPE.vi" "Focus"(w6234) -> ()
                      }
                    }
                    n3259 = property on="Hit Graph" class="IntGraph (strict)"("Z Scale.Range:Minimum"=1.0, "Z Scale.Range:Maximum"="Scale") -> ()  [unwired: 2 in, 2 out]
                    n3260 = local read "stop 2"() -> (w6158:bool)
                    n3261 = local read "End experiment"() -> (w6148:bool)
                    n3262 = Tick Count (ms)() -> (millisecond timer value=w6143:u32)
                    n3263 = Compound Arithmetic op=OR(w6158, w6157, w6154, w6153, w6152, w6151, w6150, w6148) -> (w6149:bool)
                    n3264 = local write "Focus"(w6099) -> ()
                  }
                }
                frame 1 {
                  # "Frame scan FScope"
                  n3265 = Initialize Array(u8 0 ("element"), w6285, w6286) -> (w6292:u8[][])
                  n3266 = Tick Count (ms)() -> (millisecond timer value=w6310:u32)
                  n3267 = To Unsigned Long Integer(number=w6284) -> (unsigned 32bit integer=w6283:u32[][])
                  n3268 = Unbundle By Name(w6309) -> ("status"=w6307:bool)
                  n3269 = Unbundle By Name(w6308) -> ("status"=w6306:bool)
                  n3270 = Unbundle By Name(w6305) -> ("status"=w6304:bool)
                  n3271 = while {
                    tunnel: w6318 -> [w6408]
                    tunnel: w6317 -> [w6407]
                    tunnel: [w6406] -> w6316
                    tunnel: [w6395] -> w6315
                    shift-right: [w6369] -> _
                    shift-left: w6284 -> [w6364]
                    shift-right: [w6368] -> _
                    shift-left: w6284 -> [w6363]
                    tunnel: [w6400] -> w6312
                    tunnel: w6314 -> [w6400]
                    tunnel: [w6396] -> w6311
                    tunnel: w6313 -> [w6396]
                    shift-right: [w6386] -> _
                    shift-left: w6310 -> [w6387]
                    shift-right: [w6370] -> _
                    shift-left: w6283 -> [w6365]
                    tunnel: w6307 -> [w6392]
                    tunnel: w6306 -> [w6397]
                    tunnel: w6304 -> [w6372]
                    shift-right: [w6382] -> _
                    shift-left: sgl 0.0 ("millisecond timer value") -> [w6385]
                    tunnel: w6302 -> [w6381]
                    shift-right: [w6376] -> _
                    shift-left: sgl 1.0 ("millisecond timer value") -> [w6328]
                    tunnel: w6299 -> [w6379]
                    tunnel: [w6379] -> w6297
                    tunnel: [w6378] -> w6296
                    tunnel: w6298 -> [w6378]
                    shift-right: [w6366] -> _
                    shift-left: sgl 0.0 ("millisecond timer value") -> [w6367]
                    shift-right: [w6360] -> w6280
                    shift-left: w6292 -> [w6362]
                    shift-right: [w6359] -> w6279
                    shift-left: w6292 -> [w6361]
                    tunnel: w6291 -> [w6333]
                    shift-right: [w6349] -> _
                    shift-left: w6289 -> [w6351]
                    shift-right: [w6347] -> _
                    shift-left: w6290 -> [w6348]
                    tunnel: [w6326] -> w6281
                    i -> [w6331]
                    stop <- w6391 stop-if-true
                    n3272 = local read "ScaleCluster"() -> (w6358:T3)
                    n3273 = local read "Overlay Images"() -> (w6403:bool)
                    n3274 = Bundle("ScaleCluster"=w6358, "scans to read"=w6333) -> (w6349:T20)  [unwired: 1 in]
                    n3275 = call-poly <vilib>:"DAQmx Read (Digital 1D U32 1Chan NSamp).vi"("task/channels in"=w6408, "number of samples per channel"=w6333, "error in"=w6407) -> ("task out"=w6406:refnum<k21>, "data"=w6325:u32[], "error out"=w6395:errorcluster)  [unwired: 10 in]
                    n3276 = Not Equal?(x=w6349, y=w6351) -> (x != y?=w6350:bool)
                    n3277 = call-poly <vilib>:"Ramp Pattern.vi"("start"=0.0, "end"=6.283185307179586, "samples"=w6333) -> ("Ramp Pattern"=w6342:dbl[])  [unwired: 7 in, 1 out]
                    n3278 = case shown="True" w6350 {
                      tunnel: w6381 -> [_ w6412]
                      tunnel: [w6409 w6411] -> w6347
                      tunnel: w6349 -> [_ w6410]
                      tunnel: w6348 -> [w6409 _]
                      frame False {
                      }
                      frame True {
                        n3279 = call "ScaleScanlineFScope.vi"("Parameters"=w6412, "ScaleCluster"=w6410) -> ("ScanlineScaled"=w6411:dbl[][])
                      }
                    }
                    n3280 = Split Number(x=w6325) -> (hi(x)=w6405:u16[])  [unwired: 1 out]
                    n3281 = Sine(x=w6342) -> (sin(x)=w6340:dbl[])
                    n3282 = Split Number(x=w6405) -> (hi(x)=w6343:u8[], lo(x)=w6404:u8[])
                    n3283 = case shown="False" w6403 {
                      tunnel: w6343 -> [w6446 w6465]
                      tunnel: [w6446 w6448] -> w6389
                      tunnel: w6404 -> [w6445 w6467]
                      tunnel: [w6445 _] -> w6388
                      frame False {
                      }
                      frame True {
                        n3284 = To Word Integer(number=w6465) -> (16bit integer=w6466:i16[])
                        n3285 = Subtract(x=w6466, y=w6467) -> (x-y=w6447:i16[])
                        n3286 = Add(x=w6466, y=w6467) -> (x+y=w6461:i16[])
                        n3287 = Increment(x=w6461) -> (x+1=w6471:i16[])
                        n3288 = Divide(x=w6447, y=w6471) -> (x/y=w6470:dbl[])
                        n3289 = Absolute Value(x=w6447) -> (abs(x)=w6463:i16[])
                        n3290 = Multiply(x=w6470, y=u8 2) -> (x*y=w6468:dbl[])
                        n3291 = Round To Nearest(number=w6468) -> (nearest integer value=w6454:dbl[])
                        n3292 = Divide(x=w6463, y=2.0) -> (x/y=w6460:dbl[])
                        n3293 = Divide(x=w6461, y=2.0) -> (x/y=w6459:dbl[])
                        n3294 = Add(x=w6460, y=w6459) -> (x+y=w6457:dbl[])
                        n3295 = Divide(x=w6457, y=5.0) -> (x/y=w6456:dbl[])
                        n3296 = Round To Nearest(number=w6456) -> (nearest integer value=w6455:dbl[])
                        n3297 = Multiply(x=5.0 ("y"), y=w6455) -> (x*y=w6453:dbl[])
                        n3298 = Add(x=w6454, y=w6453) -> (x+y=w6452:dbl[])
                        n3299 = Subtract(x=w6452, y=2.0) -> (x-y=w6449:dbl[])
                        n3300 = To Unsigned Byte Integer(number=w6449) -> (unsigned 8bit integer=w6448:u8[])
                      }
                    }
                    n3301 = Add(x=w6340, y=sgl 2.0 ("millisecond timer value")) -> (x+y=w6335:dbl[])
                    n3302 = Divide(x=u32 4294967295 ("millisecond timer value"), y=sgl 3.0) -> (x/y=w6336:sgl)
                    n3303 = Array Subset(array=w6347, index (col)=w6385, length (col)=w6333) -> (w6355:dbl[][])  [unwired: 2 in]
                    n3304 = Multiply(x=w6336, y=w6335) -> (x*y=w6334:dbl[])
                    n3305 = To Unsigned Long Integer(number=w6334) -> ()  [unwired: 1 out]
                    n3306 = Index Array(array=w6347, index (row)=0) -> (element=w6356:dbl[])  [unwired: 1 in]
                    n3307 = Array Size(array=w6356) -> (size(s)=w6353:i32)
                    n3308 = Divide(x=w6353, y=2) -> (x/y=w6352:dbl)
                    n3309 = Add(x=w6385, y=w6333) -> (x+y=w6383:dbl)
                    n3310 = Greater Or Equal?(x=w6383, y=w6352) -> (x >= y?=w6384:bool)
                    n3311 = case shown="True" w6384 {
                      tunnel: w6383 -> [w6441 w6444]
                      tunnel: [w6441 w6442] -> w6382
                      tunnel: w6352 -> [_ w6443]
                      frame False {
                      }
                      frame True {
                        n3312 = Subtract(x=w6444, y=w6443) -> (x-y=w6442:dbl)
                      }
                    }
                    n3313 = Multiply(x="Averaging", y="Number of Frames") -> (x*y=w6374:sgl)
                    n3314 = Tick Count (ms)() -> (millisecond timer value=w6402:u32)
                    n3315 = Decrement(x=w6374) -> (x-1=w6373:sgl)
                    n3316 = Equal?(x="Averaging", y=w6328) -> (x = y?=w6377:bool)
                    n3317 = local read "Image Update [ms]"() -> (w6399:u32)
                    n3318 = Equal?(x=w6373, y=w6331) -> (x = y?=w6371:bool)
                    n3319 = call "AverageImageFScope.vi"("HitsArray"=w6365, "ScanLineFScope"=w6355, "Image1Array"=w6364, "Image2Array"=w6363, "DataImage2"=w6388, "DataImage1"=w6389) -> ("HitsArraynew"=w6346:u32[][], "Image1Arraynew"=w6345:u8[][], "Image2Arraynew"=w6344:u8[][])
                    n3320 = Subtract(x=w6402, y=w6387) -> (x-y=w6401:u32)
                    n3321 = Increment(x=w6331) -> (x+1=w6330:i32)
                    n3322 = Greater Or Equal?(x=w6401, y=w6399) -> ()  [unwired: 1 out]
                    n3323 = Divide(x=w6330, y="Averaging") -> (x/y=w6327:sgl)
                    n3324 = local write "Hit Graph"(w6346) -> ()
                    n3325 = local write "Image 1"(w6345) -> ()
                    n3326 = local write "Image 2"(w6344) -> ()
                    n3327 = case shown="True" w6377 {
                      tunnel: w6344 -> [w6420 w6424]
                      tunnel: w6345 -> [w6419 w6429]
                      tunnel: w6346 -> [w6418 w6437]
                      tunnel: [w6418 w6436] -> w6370
                      tunnel: [w6419 w6435] -> w6369
                      tunnel: [w6420 w6434] -> w6368
                      tunnel: [w6416 sgl 1.0 ("millisecond timer value")] -> w6376
                      tunnel: w6328 -> [w6417 _]
                      tunnel: w6367 -> [w6415 w6431]
                      tunnel: [w6415 w6432] -> w6366
                      tunnel: w6362 -> [w6414 w6428]
                      tunnel: w6361 -> [w6413 w6426]
                      tunnel: [w6414 w6427] -> w6360
                      tunnel: [w6413 w6425] -> w6359
                      frame False {
                        n3328 = Increment(x=w6417) -> (x+1=w6416:sgl)
                      }
                      frame True {
                        n3329 = local read "Y dim"() -> (w6430:sgl)
                        n3330 = Multiply(x=w6430, y=w6431) -> (x*y=w6423:sgl)
                        n3331 = Multiply(x=w6424, y=u8 0 ("millisecond timer value")) -> (x*y=w6434:u8[][])
                        n3332 = Multiply(x=u8 0 ("millisecond timer value"), y=w6437) -> (x*y=w6436:u32[][])
                        n3333 = Increment(x=w6431) -> (x+1=w6432:sgl)
                        n3334 = Replace Array Subset(array=w6428, new element=w6429, index (row)=0 ("disabled index (row)"), index (col)=w6423) -> (w6427:u8[][])
                        n3335 = Replace Array Subset(array=w6426, new element=w6424, index (row)=0 ("disabled index (row)"), index (col)=w6423) -> (w6425:u8[][])
                        n3336 = Multiply(x=w6429, y=u8 0 ("millisecond timer value")) -> (x*y=w6435:u8[][])
                      }
                    }
                    n3337 = Round Toward +Infinity(x=w6327) -> (ceil(x): smallest int >= x=w6326:sgl)
                    "#" <- w6326
                    n3338 = Unbundle By Name(w6396) -> ("status"=w6394:bool)
                    n3339 = Tick Count (ms)() -> (millisecond timer value=w6386:u32)
                    n3340 = Unbundle By Name(w6378) -> ("status"=w6380:bool)
                    n3341 = Unbundle By Name(w6395) -> ("status"=w6393:bool)
                    n3342 = local read "stop 2"() -> (w6398:bool)
                    n3343 = local read "End experiment"() -> (w6390:bool)
                    n3344 = Compound Arithmetic op=OR(w6398, w6397, w6394, w6393, w6392, w6380, w6371, w6372, w6390) -> (w6391:bool)
                    "#" <- w6328
                  }
                  n3345 = Decrement(x=w6281) -> (x-1=w6282:sgl)
                }
